vi "Read_Camera.vi"(0 "error in":errorcluster, 2 "Camera":T3, 3 "node":string) -> (1 "error out":errorcluster, 4 "image data":T1)   [LabVIEW 2012]
doc: "Get an image from one of Baxter's hand cameras. \n\nIf you are running 1.1.0 or higher and reading an image in from the head camera, you must first close a hand camera and then open the head camera, waiting 5 s for each process to run.\n\nIt is highly recommended that you are connected to baxter via ethernet rather than over wireless when doing this."
uses:
  <userlib>/ROS for LabVIEW Software/ROS/Code/SubVIs/BaxterCamera.ctl
  <vilib>/picture/picture.llb/imagedata.ctl
  <userlib>/ROS for LabVIEW Software/ROS/Code/Console/Servers/ServerSubs/TopicDef.ctl
  <userlib>/ROS for LabVIEW Software/ROS/Code/SubVIs/_ROSDirection.ctl
panel:
  out "ROS Image":T2
  out "image":picture
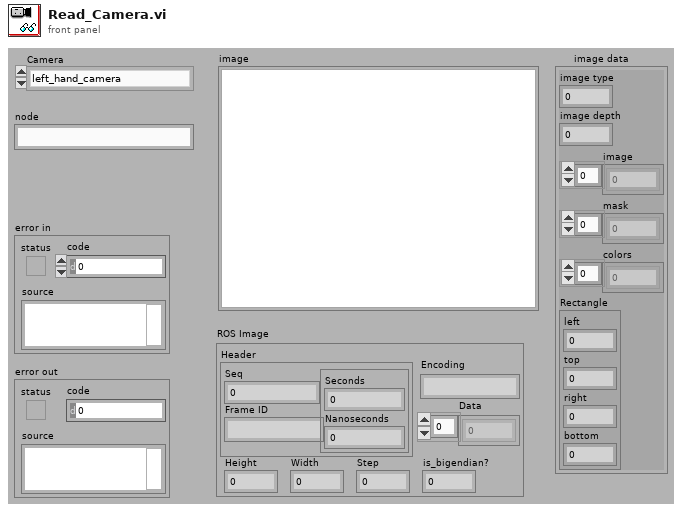
[diagram p1: front panel]
types:
  T1 = typedef "imagedata.ctl" = cluster{"image type":i32, "image depth":i32, "image":u8[], "mask":u8[], "colors":u32[], "Rectangle":cluster{"left":i16, "top":i16, "right":i16, "bottom":i16}}
  T2 = cluster{"Header":cluster{"Seq":u32, "Frame ID":string, cluster{"Seconds":i32, "Nanoseconds":i32}}, "Height":u32, "Width":u32, "is_bigendian?":u8, "Step":u32, "Data":u8[], "Encoding":string}
  T3 = typedef "BaxterCamera.ctl" = enum16{"left_hand_camera", "right_hand_camera", "head_camera"}
  T4 = typedef "TopicDef.ctl" = cluster{"Topic":string, "Type":string, "Action":T5, "Update (ms)":u16, "queue size":u16}
  T5 = typedef "_ROSDirection.ctl" = enum16{"Node", "Publisher", "Subscriber", "ServiceClient", "ServiceProvider"}
  T6 = typedef "_ROSControl.ctl" = cluster{"topic port":u16, "Node":string, "topic":string, "type":string, "node port":u16, "error ":errorcluster, "Direction":T5, "Update (ms)":u16, "FIFO size":u16}
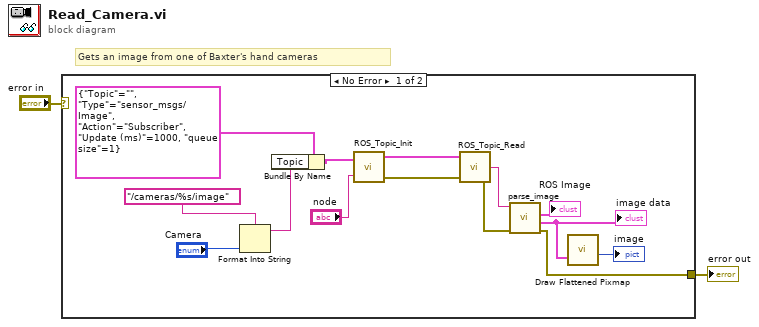
[diagram p0: block diagram]
diagram:
  # "Gets an image from one of Baxter's hand cameras"
  n1 = case shown="No Error" "error in" {
    selector: "error in" -> [_ w17]
    tunnel: [w5 w17] -> w2
    frame No Error {
      n2 = Format Into String(format string="/cameras/%s/image" ("topic"), "Camera") -> (resulting string=w11:string)  [unwired: 2 in, 1 out]
      n3 = Bundle By Name(cluster=T4 {"Topic"="", "Type"="sensor_msgs/Image", "Action"=enum."Subscriber", "Update (ms)"=1000, "queue size"=1} ("Definitions"), "Topic"=w11) -> (w10:T4)
      n4 = call <userlib>:"ROS_Topic_Init.vi"("Definitions"=w10, "node"="node") -> ("ROS out"=w15:T6, "error out"=w6:errorcluster)  [unwired: 1 in]
      n5 = call <userlib>:"ROS_Topic_Read.vi"("error in (no error)"=w6, "ROS in"=w15) -> ("error out"=w3:errorcluster, "Reply"=w4:string)  [unwired: 1 in, 1 out]
      n6 = call <userlib>:"parse_image.vi"("error in"=w3, "msg in"=w4) -> ("error out"=w5:errorcluster, "image data"=w7:T1, "ROS Image"=→"ROS Image":T2)  [unwired: 2 in, 1 out]
      "image data" <- w7
      n7 = call <vilib>:"Draw Flattened Pixmap.vi"("image data"=w7) -> ("new picture"=→"image":picture)  [unwired: 8 in]
    }
    frame Error {
    }
  }
  "error out" <- w2
